vi "Leak Test.vi"(7 "FP":T2, 8 "Results":T1[](array[typedef]), 9 "RatePass":bool[](array[boolean]), 11 "Cart Array":bool[](array[boolean])) -> (1 "Error String":string, 3 "Pass/Fail Array":bool[](array[boolean]))   [LabVIEW 2020]
uses:
  Main Refs.ctl
  Hardware/Tecan/Pump Config.ctl
  Timing Specs.ctl
  Vacuum Specs.ctl
  Cartridges.ctl
  Cartridge Status.ctl
  Commands.ctl
  Lib/Time/Wells.ctl
  Lib/Time/Bottles.ctl
  Process State.ctl
  Vacuum Test.ctl
  Vacuum Output.ctl
  Update Single Cart.ctl
panel:
  # "Tecan Pump"
  # "Pressure"
  # "General"
  # "Timing"
  # "Protocol"
  # "Zaber"
  # "NFC Reader 1"
  # "NFC  Reader 2"
  # "NFC Reader 3"
  # "NFC Reader 4"
  # "System"
  # "Cartridge Utitlies"
  # "Wells"
  # "times"
  # "from"
  # "State Machine"
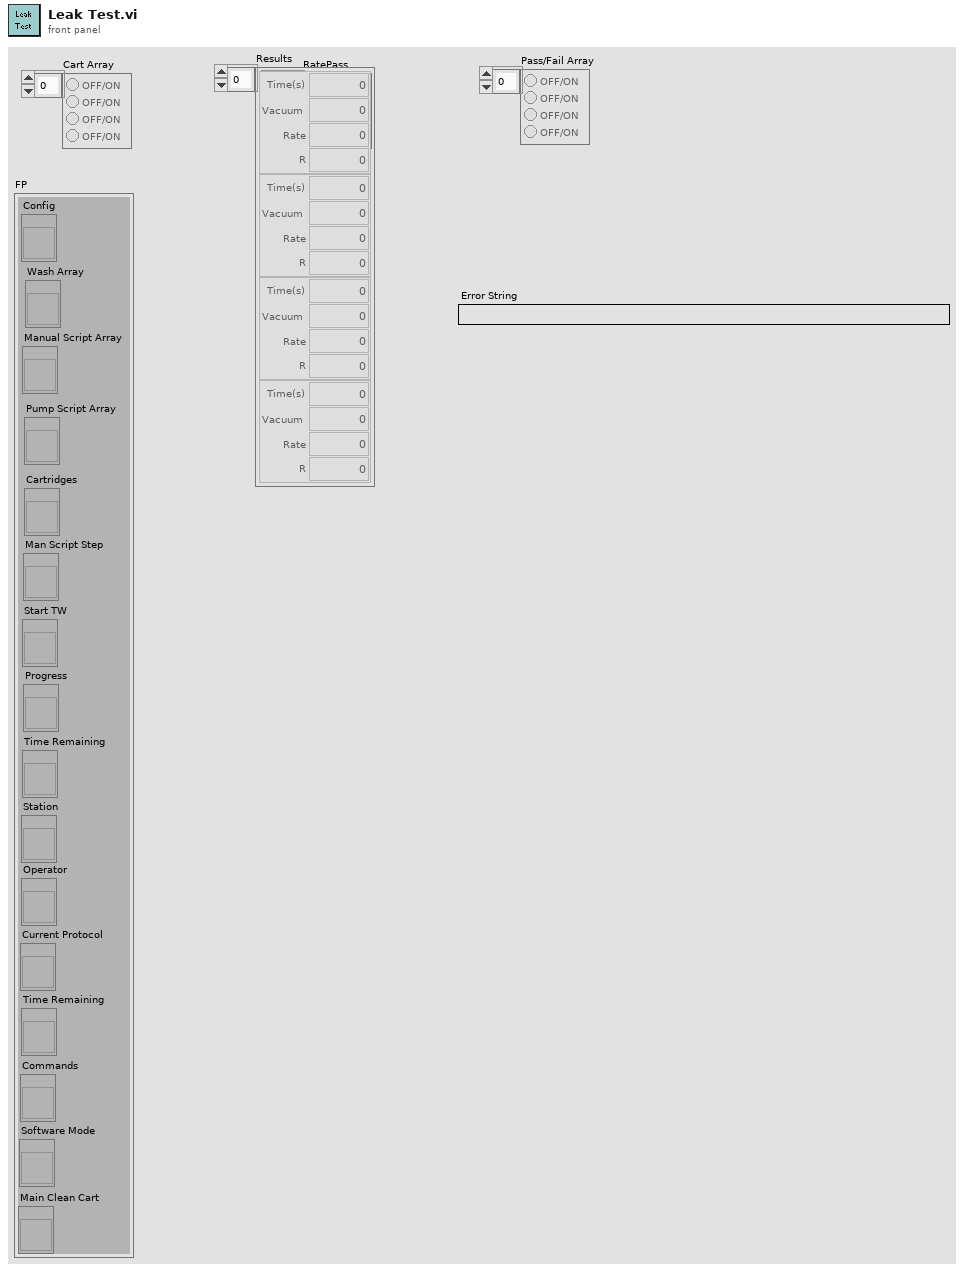
[diagram p1: front panel]
types:
  T1 = typedef "Vacuum Output.ctl" = cluster{"Time(s)":dbl, "Vacuum":dbl, "Rate":dbl, "R":dbl}
  T2 = typedef "Main Refs.ctl" = cluster{"Config":refnum<vi>, "Wash Array":refnum<vi>, "Manual Script Array":refnum<vi>, "Pump Script Array":refnum<vi>, "Cartridges":refnum<vi>, "Man Script Step":refnum<vi>, "Start TW":refnum<vi>, "Progress":refnum<vi>, "Time Remaining":refnum<vi>, "Station":refnum<vi>, "Operator":refnum<vi>, "Current Protocol":refnum<vi>, "Time Remaining":refnum<vi>, "Commands":refnum<vi>, "Software Mode":refnum<vi>, "Main Clean Cart":refnum<vi>}
  T3 = typedef "Update Single Cart.ctl" = enum16{"Cart Status", "Cart Reagent"}
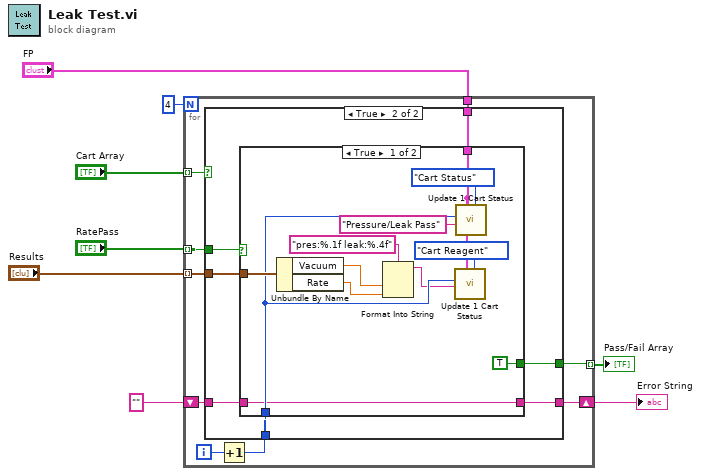
[diagram p0: block diagram]
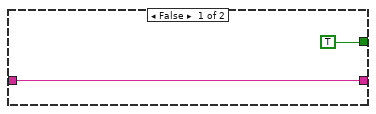
[diagram p2: hidden frame]
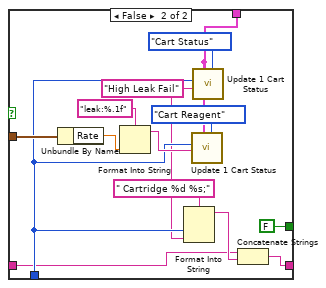
[diagram p3: hidden frame]
diagram:
  n1 = for {
    N: 4 -> [_]
    tunnel: "RatePass" -> [w16] mode=indexing
    tunnel: "Cart Array" -> [w17] mode=indexing
    tunnel: "FP" -> [w15]
    tunnel: "Results" -> [w13] mode=indexing
    shift-right: [w12] -> w7
    shift-left: "" ("String") -> [w11]
    tunnel: [w9] -> w1 mode=indexing
    i -> [w14]
    n2 = Increment(x=w14) -> (x+1=w10:i32)
    n3 = case shown="True" w17 {
      tunnel: w16 -> [_ w24]
      tunnel: w15 -> [_ w26]
      tunnel: w10 -> [_ w25]
      tunnel: w13 -> [_ w23]
      tunnel: w11 -> [w19 w22]
      tunnel: [w19 w21] -> w12
      tunnel: [TRUE w20] -> w9
      frame False {
      }
      frame True {
        n4 = case shown="True" w24 {
          tunnel: w26 -> [w32 w43]
          tunnel: w25 -> [w30 w45]
          tunnel: w23 -> [w36 w51]
          tunnel: w22 -> [w28 w41]
          tunnel: [w28 w40] -> w21
          tunnel: [TRUE FALSE] -> w20
          frame True {
            n5 = Unbundle By Name(w36) -> ("Vacuum"=w35:dbl, "Rate"=w34:dbl)
            n6 = Format Into String(format string="pres:%.1f leak:%.4f", w35, w34) -> (resulting string=w29:string)  [unwired: 2 in, 1 out]
            n7 = call "Update 1 Cart Status.vi"("Selection"=Update_Single_Cart."Cart Reagent", "FP"=w32, "String"=w29, "Cartridge"=w30) -> ()  [unwired: 7 in, 1 out]
            n8 = call "Update 1 Cart Status.vi"("Selection"=Update_Single_Cart."Cart Status", "FP"=w32, "String"="Pressure/Leak Pass", "Cartridge"=w30) -> ()  [unwired: 7 in, 1 out]
          }
          frame False {
            w44 = "High Leak Fail" ("String")
            n9 = Unbundle By Name(w51) -> ("Rate"=w47:dbl)
            n10 = Format Into String(format string="leak:%.1f", w47) -> (resulting string=w48:string)  [unwired: 2 in, 1 out]
            n11 = Format Into String(format string=" Cartridge %d %s;", w45, w44) -> (resulting string=w42:string)  [unwired: 2 in, 1 out]
            n12 = call "Update 1 Cart Status.vi"("Selection"=Update_Single_Cart."Cart Reagent", "FP"=w43, "String"=w48, "Cartridge"=w45) -> ()  [unwired: 7 in, 1 out]
            n13 = call "Update 1 Cart Status.vi"("Selection"=Update_Single_Cart."Cart Status", "FP"=w43, "String"=w44, "Cartridge"=w45) -> ()  [unwired: 7 in, 1 out]
            n14 = Concatenate Strings(w41, w42) -> (w40:string)
          }
        }
      }
    }
  }
  "Error String" <- w7
  "Pass/Fail Array" <- w1
